vi "PWM Read.vi"(8 "error in":errorcluster, 11 "FPGA Interface":refnum<k20>) -> (0 "error out":errorcluster, 1 "Frequency":dbl, 2 "Duty Cycle":dbl)   [LabVIEW 2013, in "PWM Engine.lvlib"]
uses:
  PWM Engine.lvlib
  <vilib>/rvi/interface/common/niFpgaWaitOnOcc.vi
  <vilib>/Utility/error.llb/Error Cluster From Error Code.vi
  <vilib>/rvi/errors/niLvFpgaAdjustHostInterfaceError.vi
  <vilib>/rvi/interface/nirviReadWriteControl/nirviReadWriteControl.xnode
  NiFpgaLv.dll
  <vilib>/rvi/interface/Simulation/niFpgaSimulationCallBeginRW.vi
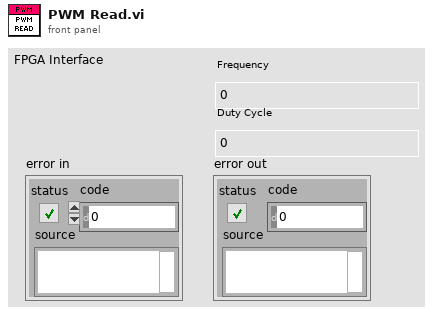
[diagram p1: front panel]
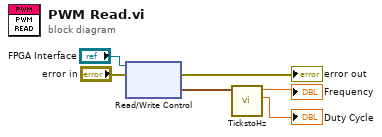
[diagram p0: block diagram]
diagram:
  n1 = xnode "Read/Write Control"("FPGA VI Reference In"="FPGA Interface", "error in"="error in") -> ("error out"=→"error out":errorcluster, "Value"=w4:cluster{"Low Ticks":u32, "High Ticks":u32})  [unwired: 1 out]
  n2 = call "TickstoHz.vi"("Ticks"=w4) -> ("Duty Cycle"=→"Duty Cycle":dbl, "Frequency"=→"Frequency":dbl)  [unwired: 9 in]
